vi "AVA Telemetry Name Reader.vi"(11 "Path":path=path "C:/Users/dgrimm/Desktop/Raw Data Files/AVA Tlm Db.txt") -> (3 "Telemetry Names":string[](array[string]))   [LabVIEW 2021]
uses:
  <vilib>/Utility/file.llb/Read Delimited Spreadsheet (string).vi
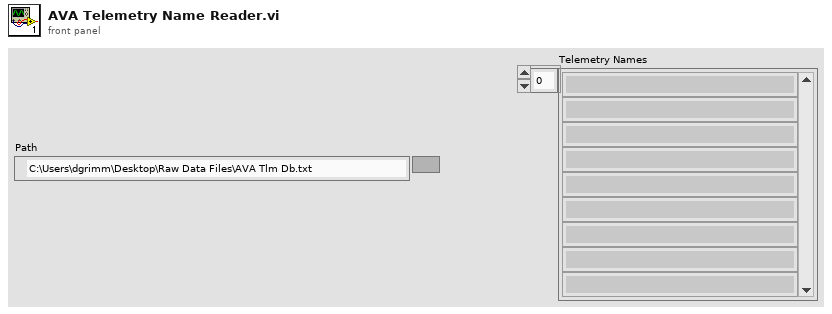
[diagram p1: front panel]
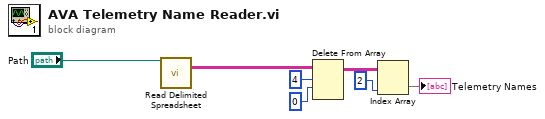
[diagram p0: block diagram]
diagram:
  n1 = call-poly <vilib>:"Read Delimited Spreadsheet.vi"("file path (dialog if empty)"="Path") -> ("all rows"=w6:string[][])  [unwired: 9 in, 5 out]
  n2 = Delete From Array(array=w6, length=4, index (row)=0 ("disabled index (col)")) -> (array with subset deleted=w3:string[][])  [unwired: 1 in, 1 out]
  n3 = Index Array(array=w3, index (col)=2 ("disabled index (col)")) -> (element=→"Telemetry Names":string[])  [unwired: 1 in]
